vi "计算短轴xy 长度.vi"(11 "Minor Axis":T1) -> (1 "短轴长度":dbl, 2 "第二点y值，x=639":dbl, 3 "第一点y值，x=0":dbl)   [LabVIEW 2015]
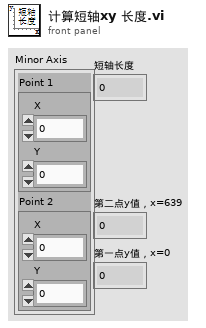
[diagram p1: front panel]
types:
  T1 = cluster{"Point 1":cluster{"X":sgl, "Y":sgl}, "Point 2":cluster{"X":sgl, "Y":sgl}}
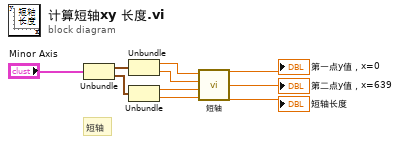
[diagram p0: block diagram]
diagram:
  # "短轴"
  n1 = Unbundle("Minor Axis") -> ("Point 1"=w10:cluster{"X":sgl, "Y":sgl}, "Point 2"=w9:cluster{"X":sgl, "Y":sgl})
  n2 = Unbundle(w10) -> ("X"=w8:sgl, "Y"=w7:sgl)
  n3 = Unbundle(w9) -> ("X"=w6:sgl, "Y"=w5:sgl)
  n4 = call "短轴.vi"("y2"=w5, "x2"=w6, "y1"=w7, "x1"=w8) -> ("短轴长度"=→"短轴长度":dbl, "第二点y值，x=639"=→"第二点y值，x=639":dbl, "第一点y值，x=0"=→"第一点y值，x=0":dbl)  [unwired: 5 in]
